vi "Get Button Refnums.vi"(8 "error in (no error)":errorcluster, 11 "Basic Form in":refnum<class "Basic Form.lvclass">) -> (0 "error out":errorcluster, 2 "Button Refnums":map{string, refnum<vi>}(c390), 3 "Basic Form out":refnum<class "Basic Form.lvclass">)   [LabVIEW 2020, in "Form.lvlib" / "Basic Form.lvclass"]
uses:
  Basic Form.lvclass
  Basic Form.lvclass/Basic Form.ctl
  Button Libraries/Button Interface Class/Button Interface.lvclass
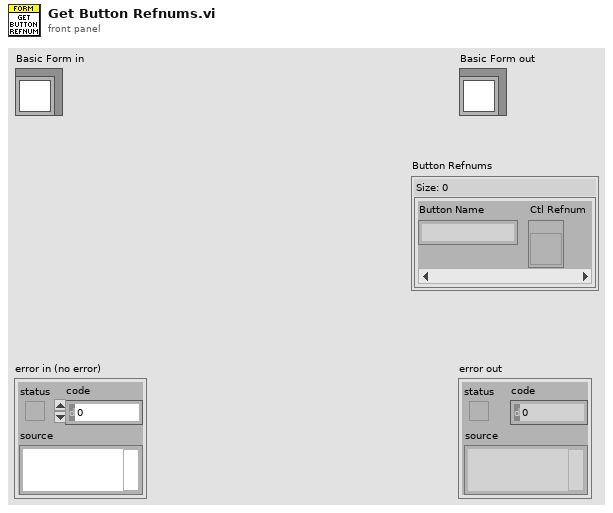
[diagram p1: front panel]
types:
  T1 = map{string, refnum<class "Button Interface.lvclass">}
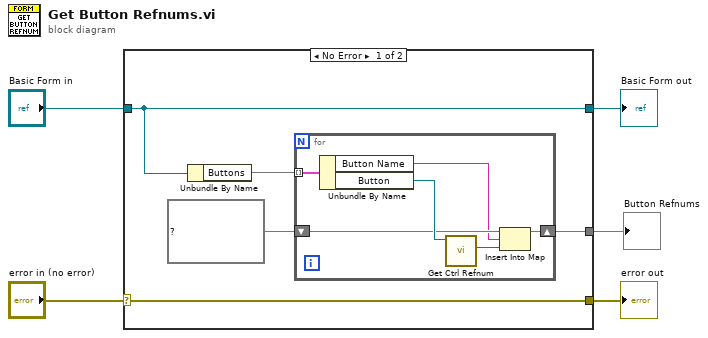
[diagram p0: block diagram]
diagram:
  n1 = case shown="No Error" "error in (no error)" {
    selector: "error in (no error)" -> [w10 w18]
    tunnel: [w10 w18] -> w4
    tunnel: [w9 w17] -> w2
    tunnel: "Basic Form in" -> [w9 w17]
    tunnel: [w6 _] -> w1
    frame No Error {
      n2 = Unbundle By Name(w9) -> ("Buttons"=w8:T1)
      n3 = for {
        tunnel: w8 -> [w16] mode=indexing
        shift-right: [w14] -> w6
        shift-left: map{string, refnum<vi>} {} ("Button Refnums") -> [w13]
        n4 = Unbundle By Name(w16) -> ("Button Name"=w11:string, "Button"=w15:refnum<class "Button Interface.lvclass">)
        n5 = call-dynamic "Get Ctrl Refnum.vi"("Button Interface in"=w15) -> ("Ctl Refnum"=w12:refnum<vi>)  [unwired: 8 in, 2 out]
        n6 = Insert Into Map(map in=w13, key=w11, value=w12) -> (map out=w14:map{string, refnum<vi>})  [unwired: 2 out]
      }
    }
    frame Error {
    }
  }
  "error out" <- w4
  "Basic Form out" <- w2
  "Button Refnums" <- w1
